vi "PJT_12.vi"() -> ()   [LabVIEW 2019]
panel:
  in  "노브":dbl(knob) scale=0.0..100.0
  out "게이지":cluster{dbl, dbl}(knob)={0.0, 8.64646225009303} scale=0.0..10.0
  in  "슬라이드":cluster{dbl, dbl}(slide)={0.0, 7.244897959183674} scale=0.0..10.0
  out "슬라이드 2":dbl(slide) scale=0.0..100.0
  out "숫자형 2":dbl
  in  "숫자형":dbl
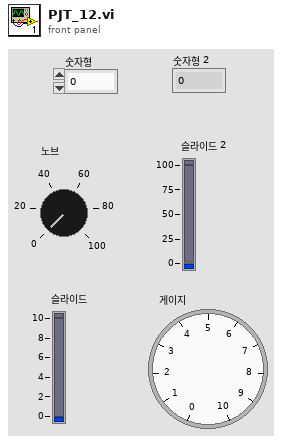
[diagram p1: front panel]
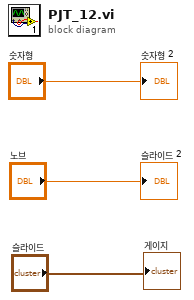
[diagram p0: block diagram]
diagram:
  "숫자형 2" <- "숫자형"
  "슬라이드 2" <- "노브"
  "게이지" <- "슬라이드"
